vi "RT_Data Convert.vi"(1 "Channel":i32, 2 "Data In":i16[](array[numeric])) -> (0 "Data Out":waveform(dbl)[](array[waveform]))   [LabVIEW 2018]
panel:
  out "Waveform Graph":dbl[](graph)
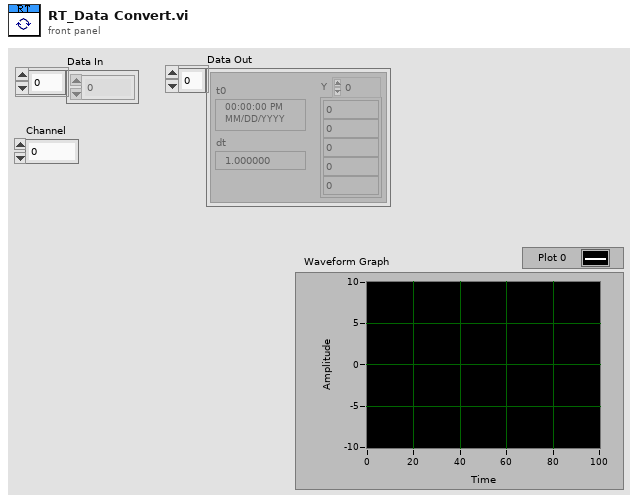
[diagram p1: front panel]
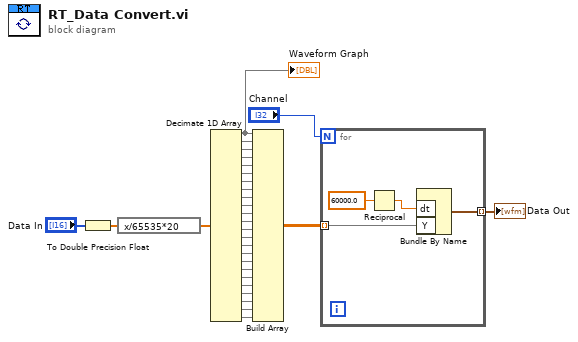
[diagram p0: block diagram]
diagram:
  n1 = To Double Precision Float(number="Data In") -> (double precision float=w30:dbl[])
  n2 = expression code="x/65535*20"(w30) -> (w28:dbl[])
  n3 = Decimate 1D Array(w28) -> (w1:dbl[], w27:dbl[], w26:dbl[], w25:dbl[], w24:dbl[], w23:dbl[], w22:dbl[], w21:dbl[], w20:dbl[], w19:dbl[], w18:dbl[], w17:dbl[], w16:dbl[], w15:dbl[], w14:dbl[], w13:dbl[], w12:dbl[], w11:dbl[], w10:dbl[], w9:dbl[], w8:dbl[], w7:dbl[], w6:dbl[], w5:dbl[])
  "Waveform Graph" <- w1
  n4 = Build Array(w1, w27, w26, w25, w24, w23, w22, w21, w20, w19, w18, w17, w16, w15, w14, w13, w12, w11, w10, w9, w8, w7, w6, w5) -> (w4:dbl[][])
  n5 = for {
    N: "Channel" -> [_]
    tunnel: w4 -> [w32] mode=indexing
    tunnel: [w31] -> w3 mode=indexing
    n6 = Reciprocal(x=60000.0) -> (1/x=w34:dbl)
    n7 = Bundle By Name("dt"=w34, "Y"=w32) -> (w31:waveform(dbl))  [unwired: 1 in]
  }
  "Data Out" <- w3
